vi "Read Config.vi"(8 "error in (no error)":errorcluster, 10 "Path to Config Folder":path, 11 "Station Config in":refnum<class "Station Config.lvclass">) -> (0 "error out":errorcluster, 3 "Station Config out":refnum<class "Station Config.lvclass">)   [LabVIEW 2017, in "Station Config.lvlib" / "Station Config.lvclass"]
doc: "Reads a recipe for a specified Material Type and stores it into memory."
uses:
  Station Config.lvclass
  <vilib>/Utility/file.llb/Read Delimited Spreadsheet (string).vi
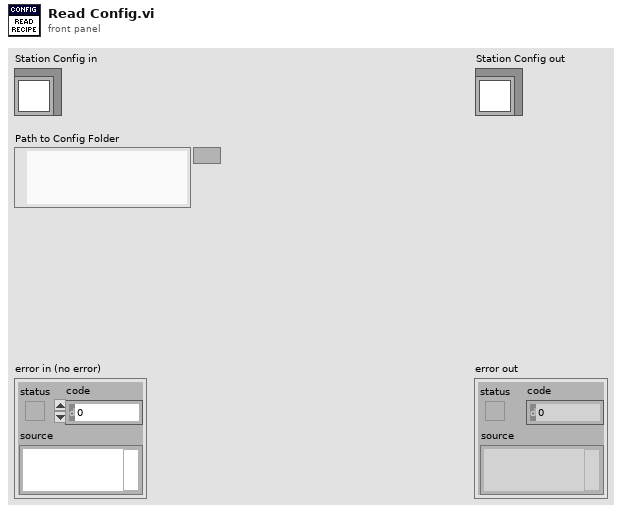
[diagram p1: front panel]
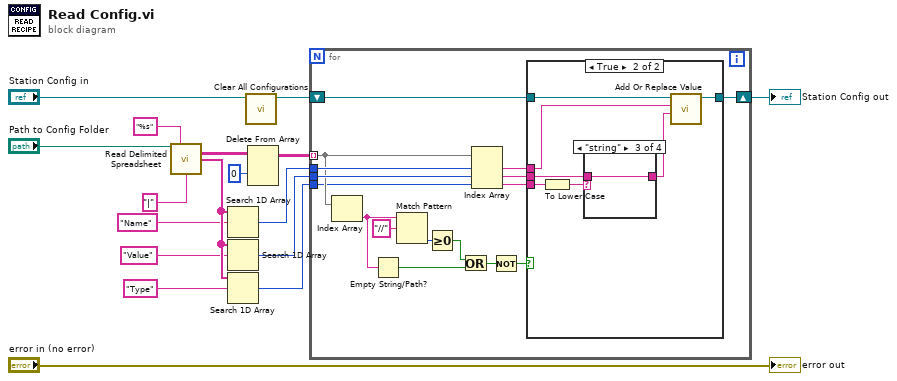
[diagram p0: block diagram]
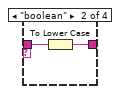
[diagram p4: hidden frame]
diagram:
  n1 = call-poly <vilib>:"Read Delimited Spreadsheet.vi"("file path (dialog if empty)"="Path to Config Folder", "format (%s)"="%s" ("format (%.3f)"), "delimiter (\\t)"="|" ("delimiter (\\t)")) -> ("all rows"=w10:string[][], "first row"=w16:string[])  [unwired: 7 in, 4 out]
  n2 = Search 1D Array(1D array=w16, element="Name") -> (index of element=w13:i32)  [unwired: 1 in]
  n3 = Search 1D Array(1D array=w16, element="Value") -> (index of element=w14:i32)  [unwired: 1 in]
  n4 = Search 1D Array(1D array=w16, element="Type") -> (index of element=w17:i32)  [unwired: 1 in]
  n5 = call "Clear All Configurations.vi"("Station Config in"="Station Config in") -> ("Station Config out"=w1:refnum<class "Station Config.lvclass">)  [unwired: 9 in, 1 out]
  n6 = Delete From Array(array=w10, index (row)=0) -> (array with subset deleted=w12:string[][])  [unwired: 2 in, 1 out]
  n7 = for {
    tunnel: w12 -> [w31] mode=indexing
    tunnel: w13 -> [w33]
    tunnel: w14 -> [w32]
    tunnel: w17 -> [w21]
    shift-right: [w18] -> w5
    shift-left: w1 -> [w19]
    n8 = Index Array(array=w31) -> (element=w29:string)  [unwired: 1 in]
    n9 = Empty String/Path?(string/path=w29) -> (empty?=w26:bool)
    n10 = Match Pattern(string=w29, regular expression="//") -> (offset past match=w27:i32)  [unwired: 1 in, 3 out]
    n11 = Greater Or Equal To 0?(x=w27) -> (x >= 0?=w25:bool)
    n12 = Or(x=w25, y=w26) -> (x .or. y?=w28:bool)
    n13 = Index Array(array=w31, index #1=w33, index #2=w32, index #3=w21) -> (element #1=w23:string, element #2=w22:string, element #3=w20:string)
    n14 = Not(x=w28) -> (.not. x?=w24:bool)
    n15 = case shown="True" w24 {
      tunnel: w23 -> [_ w37]
      tunnel: w22 -> [_ w40]
      tunnel: w20 -> [_ w41]
      tunnel: w19 -> [w34 w38]
      tunnel: [w34 w35] -> w18
      frame False {
      }
      frame True {
        n16 = To Lower Case(string=w41) -> (all lower case string=w39:string)
        n17 = case shown="\"string\"" w39 {
          tunnel: w40 -> [w42 w44 w45 w46]
          tunnel: [w42 w43 w45 w46] -> w36
          frame Default {
          }
          frame "boolean" {
            n18 = To Lower Case(string=w44) -> (all lower case string=w43:string)
          }
          frame "string" {
          }
          frame "decimal", "double", "integer", "numeric" {
          }
        }
        n19 = call-dynamic "Add Or Replace Value.vi"("Value"=w36, "Key"=w37, "Registry in"=w38) -> ("Registry out"=w35:refnum<class "Station Config.lvclass">)  [unwired: 6 in, 2 out]
      }
    }
  }
  "Station Config out" <- w5
  "error out" <- "error in (no error)"
